vi "PDLM_GetLibraryVersion.vi"(8 "error in (no error)":errorcluster) -> (0 "error out":errorcluster, 2 "Version":string, 3 "return type":i32)   [LabVIEW 2019]
uses:
  <userlib>/TaikoLaser/PDLM_DllPath_global.vi
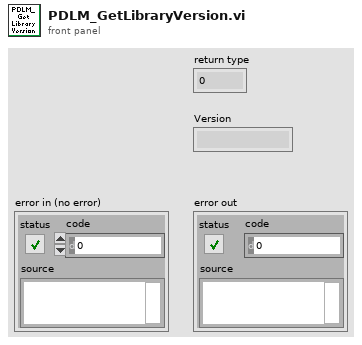
[diagram p1: front panel]
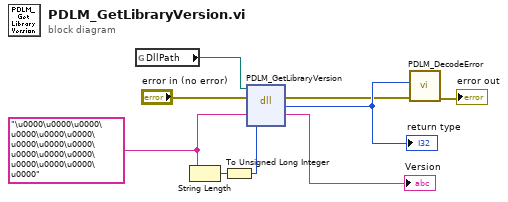
[diagram p0: block diagram]
diagram:
  w3 = "\u0000\u0000\u0000\u0000\u0000\u0000\u0000\u0000\u0000\u0000\u0000\u0000\u0000\u0000\u0000\u0000" ("Version")
  n1 = global read "PDLM_DllPath_global.vi" "DllPath"() -> (w4:path)
  n2 = String Length(string=w3) -> (length=w2:i32)
  n3 = To Unsigned Long Integer(number=w2) -> (unsigned 32bit integer=w1:u32)
  n4 = dll-call lib="M:/_dev/progs/LabVIEW/_lib/PQ/Taiko/pdlm_lib.dll" fn="PDLM_GetLibraryVersion"(path in=w4, error in="error in (no error)", "Version"=w3, "BuffLen"=w1) -> (error out=w6:errorcluster, "return type"=w7:i32, "Version"=→"Version":string)  [unwired: 2 in, 1 out]
  "return type" <- w7
  n5 = call <userlib>:"PDLM_DecodeError.vi"("error in (no error)"=w6, "code"=w7) -> ("error out"=→"error out":errorcluster)  [unwired: 7 in, 2 out]
